vi "溶解氧电极校准.vi"() -> ()   [LabVIEW 2016, in "斯坦道多参数.lvlib"]
uses:
  <vilib>/Utility/miscctls.llb/LVPointTypeDef.ctl
  <vilib>/Analysis/NI_AALBase.lvlib
panel:
  out "第二点校准值":dbl
  out "第一点校准值":dbl
  out "最小值":sgl format="%#.2f"
  out "最大值":sgl format="%#.2f"
  in  "校准模式":enum16{"两点校准", "单点校准"}(ring)=enum."单点校准"
  in  "校准停止":bool
  in  "校准启动":bool
  out "波形图表":sgl(graph) caption="历史曲线"
  out "变异系数":dbl format="%#.6f"
  out "standard deviation":dbl caption="标准差" format="%#.2f"
  out "mean":dbl caption="均值" format="%#.2f"
  out "测量读值":dbl
  out "偏移值补偿":dbl
  out "饱和度值":dbl
  out "提示":string
  out "气压补偿值":dbl
  out "盐度补偿值":dbl
  out "电极斜率":dbl
  out "电极零点":dbl
  # "溶解氧电极设定"
  # "%"
  # "%"
  # "%"
  # "mg/L"
  # "ppt"
  # "hPa"
  # "mg/L"
  # "请选择校准模式:"
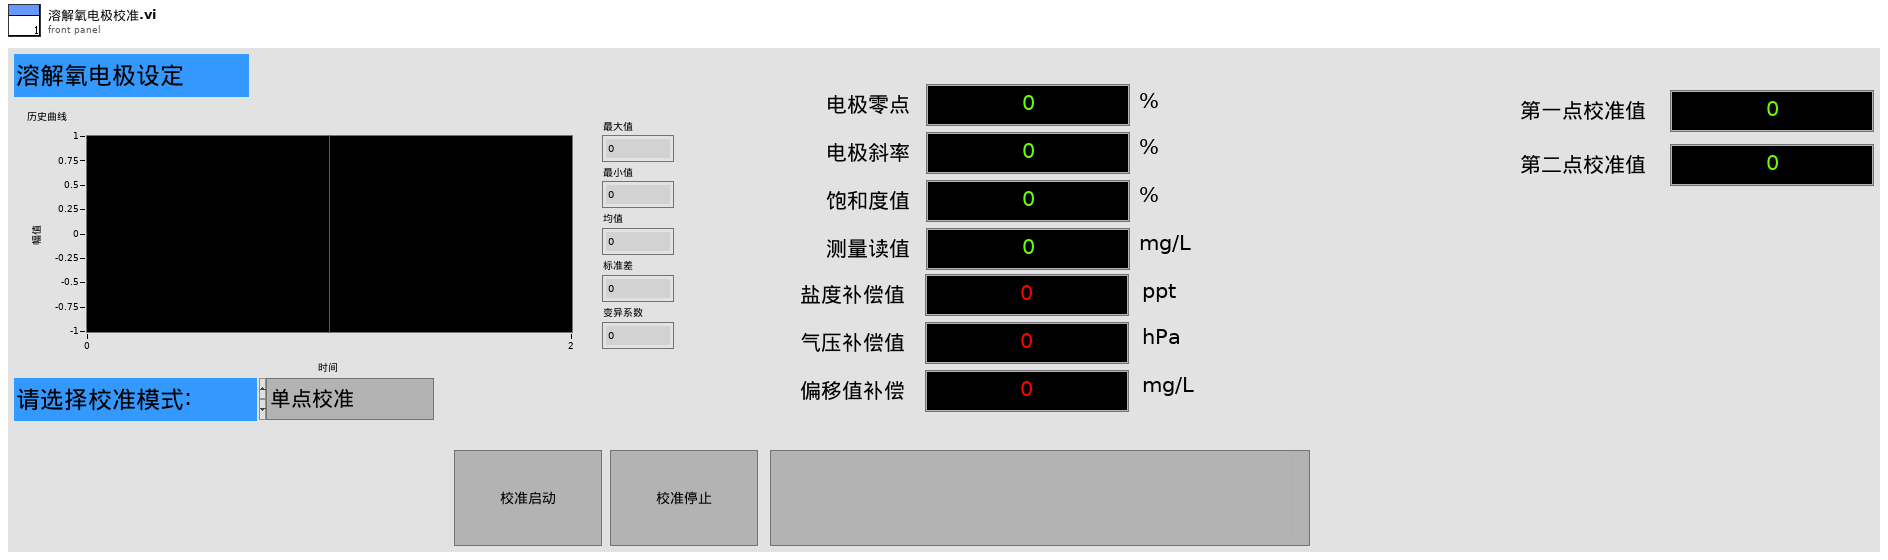
[diagram p1: front panel]
types:
  T1 = typedef "斯坦道多参数.lvlib/校准步骤.ctl" = enum16{"待机", "放置第一点标液", "第一点校准启动", "第一点校准写入", "第一点校准失败", "放置第二点标液", "第二点校准启动", "第二点校准写入", "第二点校准失败", "放置第三点标液", "第三点校准启动", "第三点校准写入", "第三点校准失败", "校准结果写入", "校准结束"}
  T2 = typedef "LVPointTypeDef.ctl" = cluster{"Horizontal":i16, "Vertical":i16}
  T3 = cluster{"电极状态标志":u16, "电极型号标志":u16, "溶解氧测量值":sgl, "温度测量值":sgl, "溶解氧饱和度值":sgl, "盐度补偿值":sgl, "大气压补偿值":sgl, "溶解氧偏移修正值":sgl, "温度偏移修正值":sgl, "手动温度补偿值":sgl, "溶解氧电极零点":sgl, "溶解氧电极斜率":sgl, "第1点标准值记录":sgl, "第1点信号值记录":sgl, "第1点温度值记录":sgl, "第2点标准值记录":sgl, "第2点信号值记录":sgl, "第2点温度值记录":sgl, "命令滤波设定":u16, "温度模式":enum16{"ATC", "MTC"}, "生产批次":u16, "电极序号":u16, "串口地址":u16, "串口波特率":enum16{"9600", "19200", "115200"}, "串口校验位":enum16{"NONE", "ODD", "EVEN"}, "串口停止位":enum16{"1bit", "2bit"}, "第一点标准值":sgl, "第二点标准值":sgl}
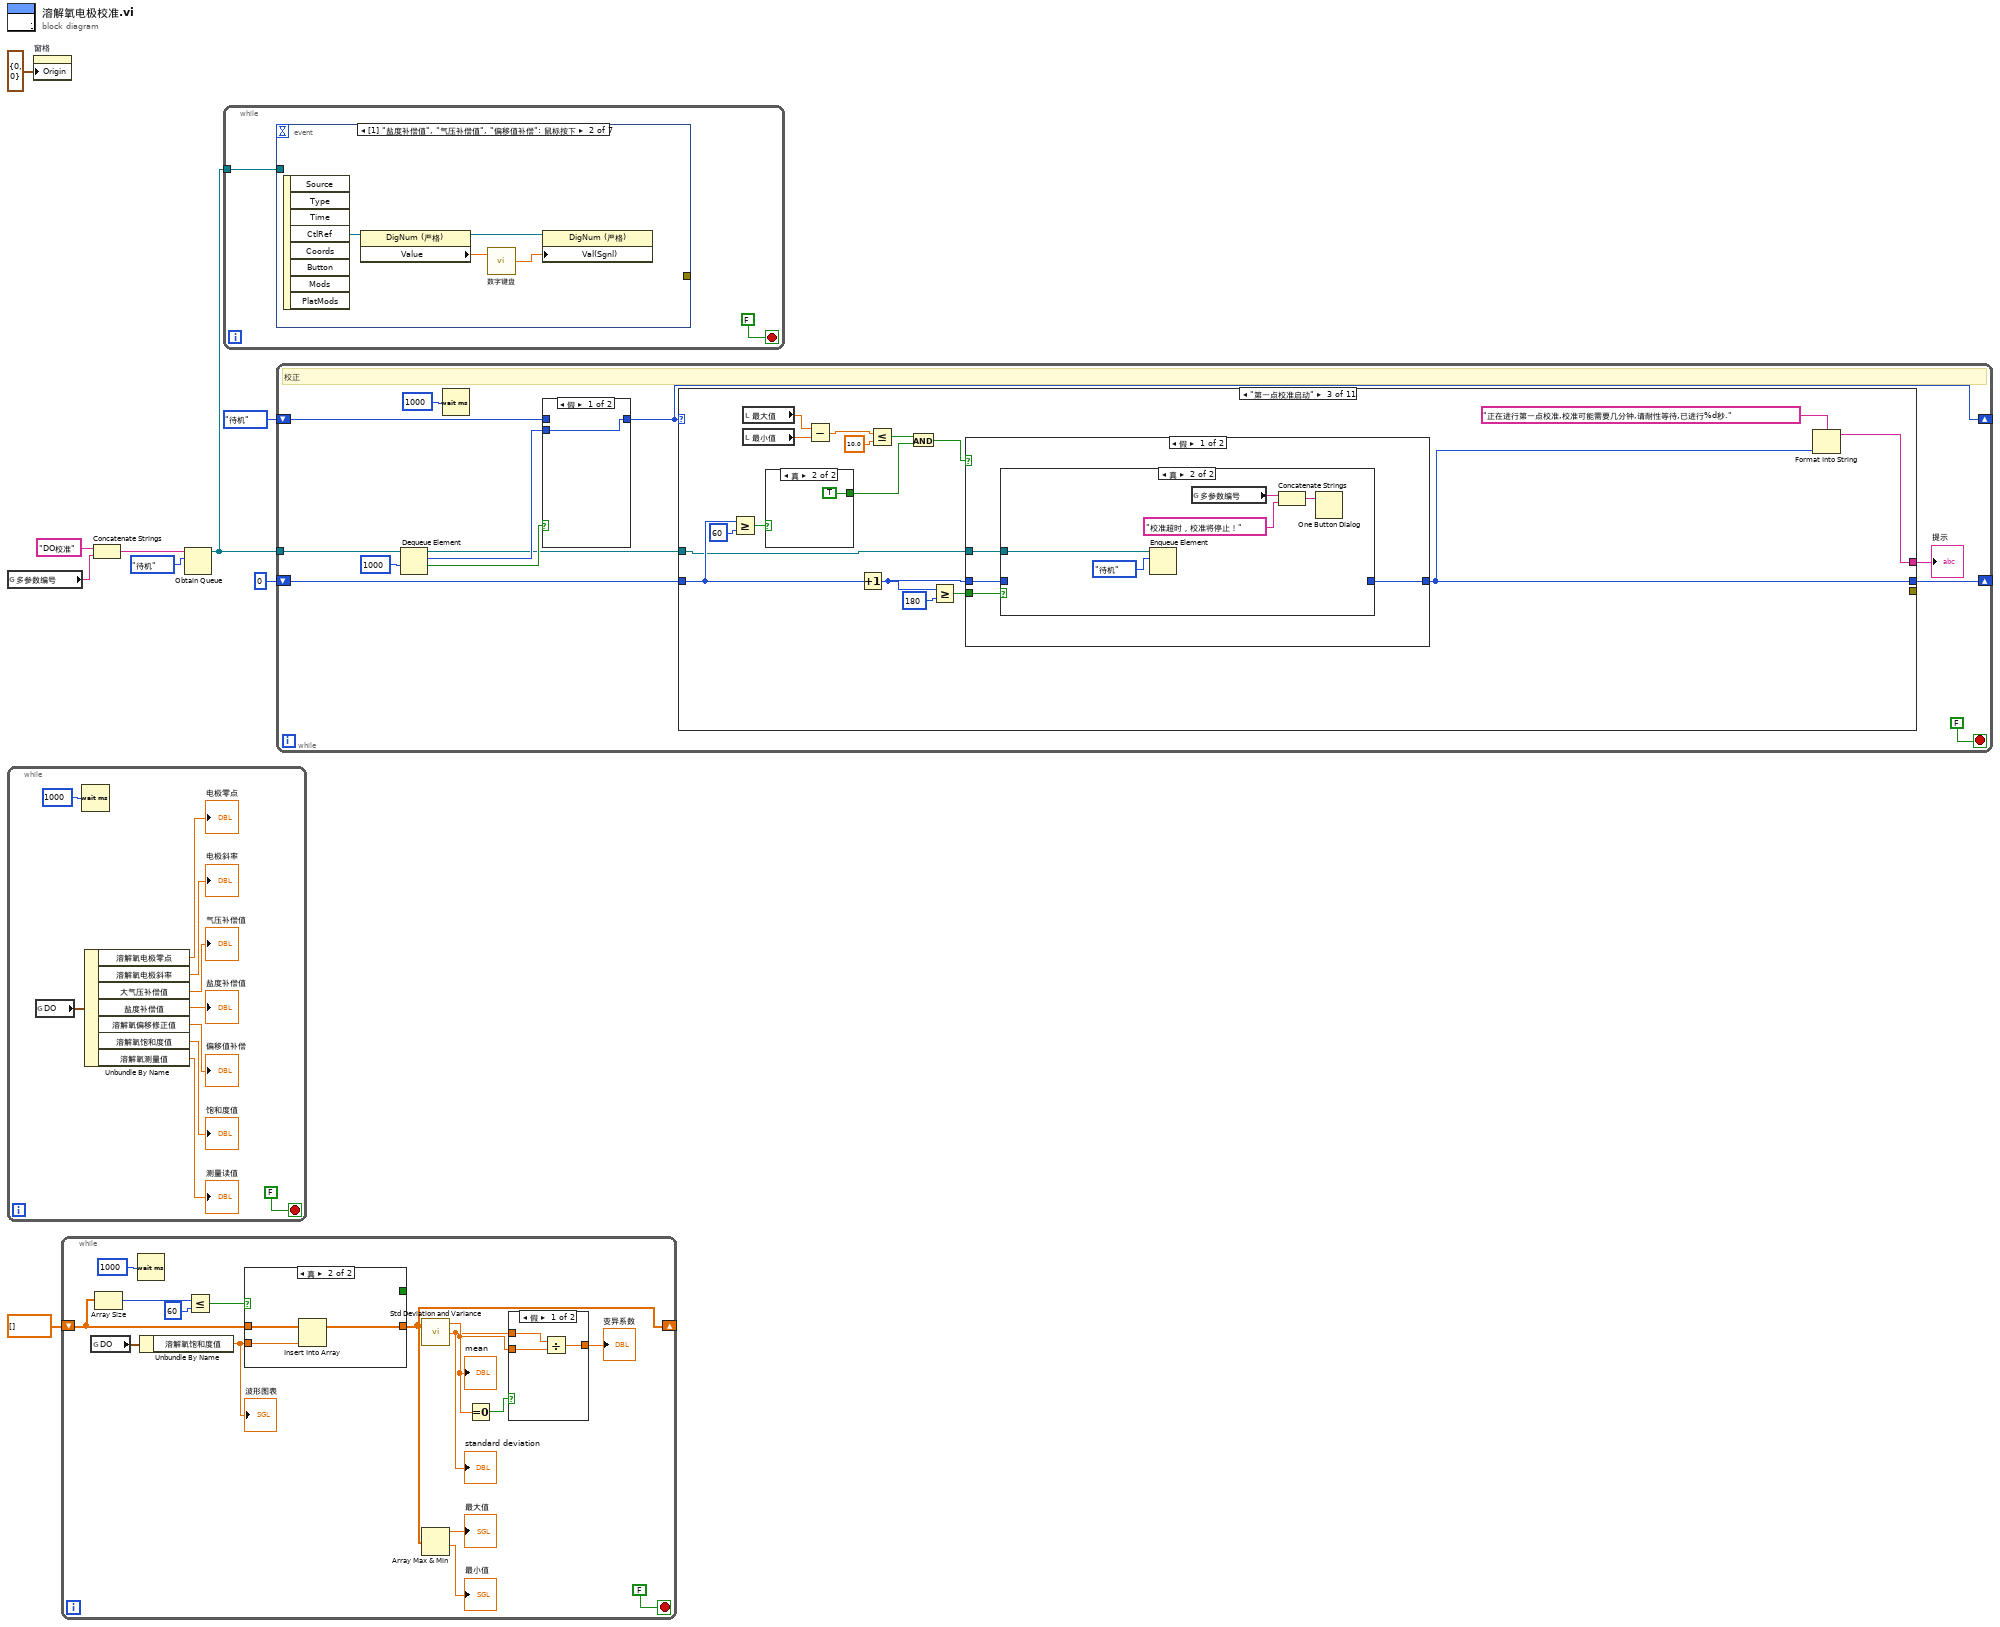
[diagram p0: block diagram]
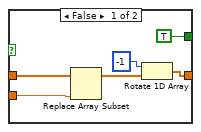
[diagram p3: hidden frame]
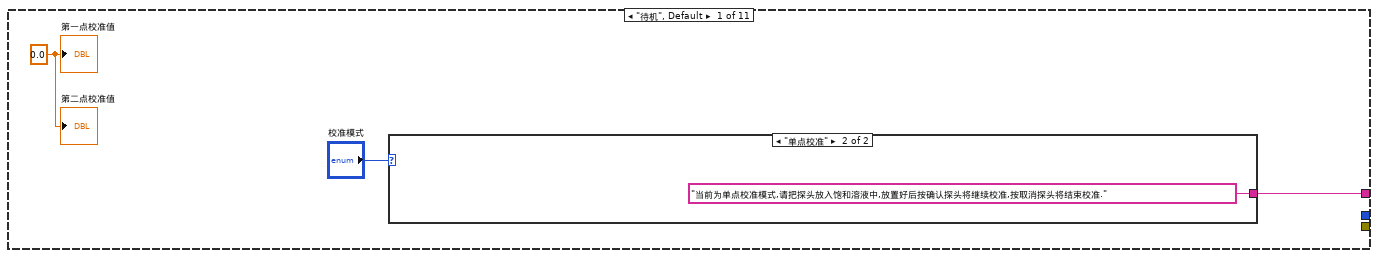
[diagram p5: hidden frame]
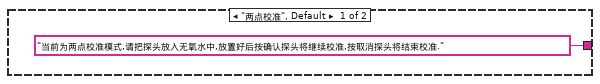
[diagram p6: hidden frame]
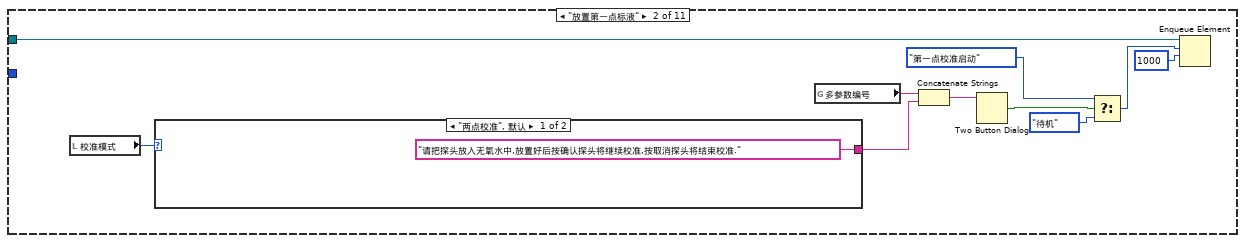
[diagram p7: hidden frame]
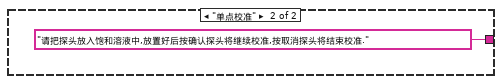
[diagram p8: hidden frame]
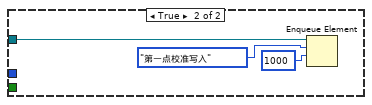
[diagram p10: hidden frame]
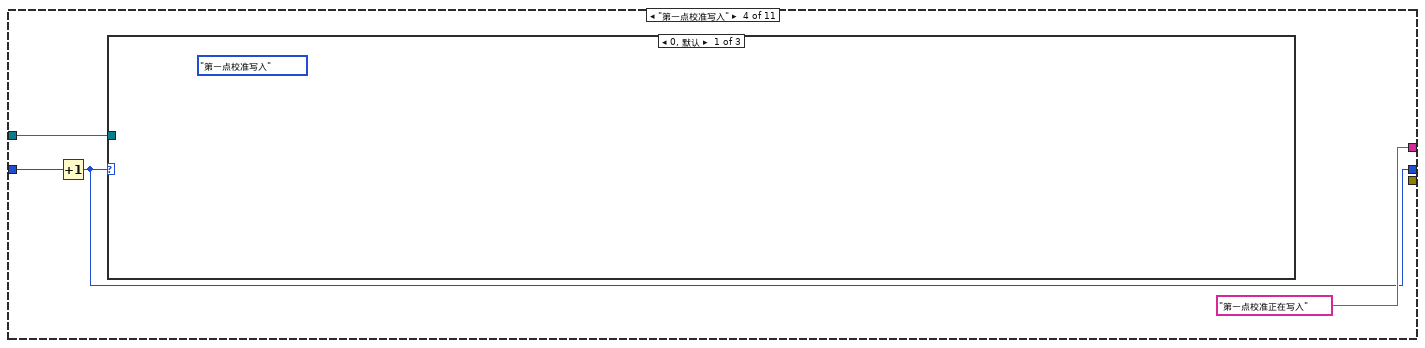
[diagram p12: hidden frame]
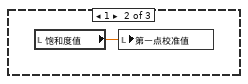
[diagram p13: hidden frame]
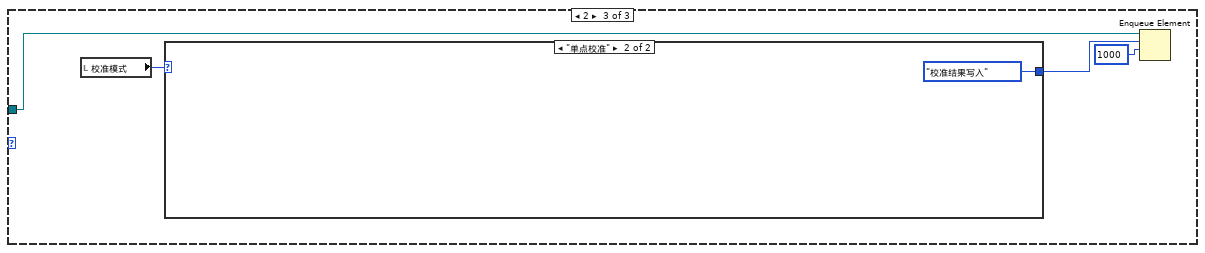
[diagram p14: hidden frame]
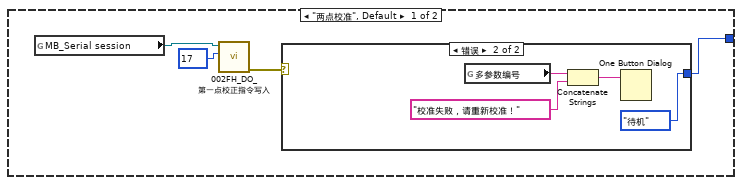
[diagram p15: hidden frame]
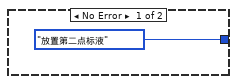
[diagram p16: hidden frame]
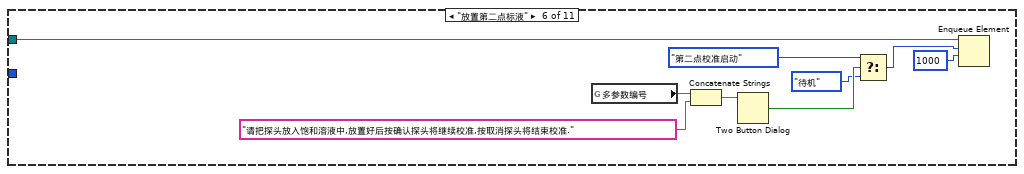
[diagram p18: hidden frame]
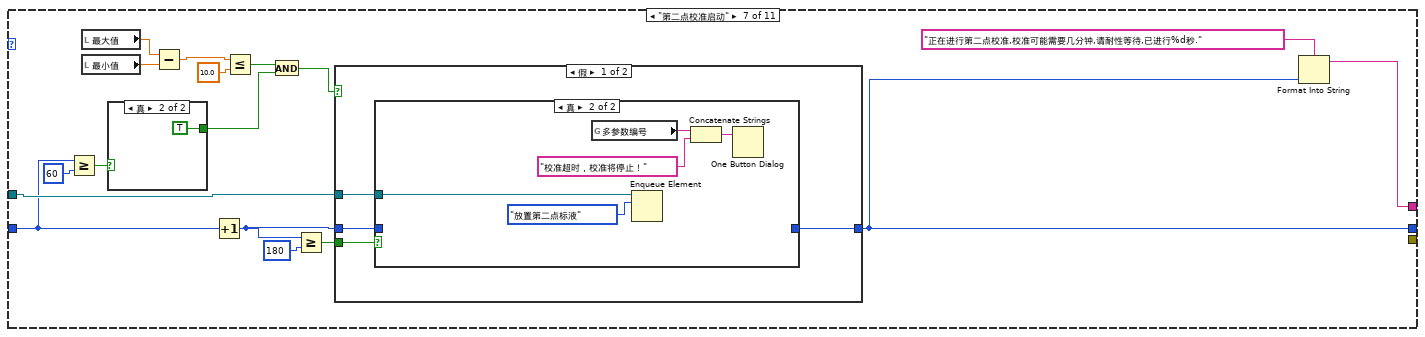
[diagram p19: hidden frame]
diagram:
  n1 = global read "多参数全局变量.vi" "多参数编号"() -> (w1:string)
  n2 = while {
    stop <- FALSE stop-if-true
    n3 = global read "国弘过程全局变量.vi" "DO"() -> (w17:T3)
    n4 = Wait (ms)(milliseconds to wait=u32 1000 ("等待时间（毫秒）")) -> ()  [unwired: 1 out]
    n5 = Unbundle By Name(w17) -> ("溶解氧电极零点"=→"电极零点":sgl, "溶解氧电极斜率"=→"电极斜率":sgl, "大气压补偿值"=→"气压补偿值":sgl, "盐度补偿值"=→"盐度补偿值":sgl, "溶解氧偏移修正值"=→"偏移值补偿":sgl, "溶解氧饱和度值"=→"饱和度值":sgl, "溶解氧测量值"=→"测量读值":sgl)
  }
  n6 = property on="窗格" class="Pane"("Origin"=T2 {"Horizontal"=0, "Vertical"=0} ("原点")) -> ()  [unwired: 2 in, 2 out]
  n7 = while {
    shift-right: [w23] -> _
    shift-left: sgl[] [] -> [w30]
    stop <- FALSE stop-if-true
    n8 = global read "国弘过程全局变量.vi" "DO"() -> (w26:T3)
    n9 = Array Size(array=w30) -> (size(s)=w32:i32)
    n10 = Wait (ms)(milliseconds to wait=u32 1000 ("等待时间（毫秒）")) -> ()  [unwired: 1 out]
    n11 = Unbundle By Name(w26) -> ("溶解氧饱和度值"=w20:sgl)
    "波形图表" <- w20
    n12 = Less Or Equal?(x=w32, y=60) -> (x <= y?=w31:bool)
    n13 = case shown="真" w31 {
      tunnel: w30 -> [w43 w46]
      tunnel: w20 -> [w41 w45]
      tunnel: [w39 w44] -> w23
      tunnel: [TRUE _] -> _
      frame False {
        n14 = Replace Array Subset(array=w43, new element=w41) -> (w42:sgl[])  [unwired: 1 in]
        n15 = Rotate 1D Array(1:w42, 2:-1 ("n")) -> (0:w39:sgl[])
      }
      frame True {
        n16 = Insert Into Array(array=w46, new element=w45) -> (w44:sgl[])  [unwired: 1 in]
      }
    }
    n17 = call <vilib>:"Std Deviation and Variance.vi"("X"=w23) -> ("mean"=w25:dbl, "standard deviation"=w24:dbl)  [unwired: 1 in, 1 out]
    "mean" <- w25
    "standard deviation" <- w24
    n18 = Array Max & Min(array=w23) -> (max value=→"最大值":sgl, min value=→"最小值":sgl)  [unwired: 2 out]
    n19 = Equal To 0?(x=w25) -> (x = 0?=w29:bool)
    n20 = case shown="假" w29 {
      tunnel: w24 -> [w37 _]
      tunnel: [w36 _] -> w28
      tunnel: w25 -> [w35 _]
      frame False {
        n21 = Divide(x=w37, y=w35) -> (x/y=w36:dbl)
      }
      frame True {
      }
    }
    "变异系数" <- w28
  }
  n22 = Concatenate Strings("DO校准" ("名称（未命名）"), w1) -> (w2:string)
  n23 = Obtain Queue(name (unnamed)=w2, element data type=校准步骤."待机" ("枚举")) -> (queue out=w3:refnum<queue>)  [unwired: 3 in, 2 out]
  n24 = while {
    tunnel: w3 -> [w47]
    stop <- FALSE stop-if-true
    n25 = event shown="[1] \"盐度补偿值\", \"气压补偿值\", \"偏移值补偿\": 鼠标按下" {
      selector: _ -> [_ _ _ _ _ _ _]
      dyn-events: _ -> [_ _ _ _ _ _ _]
      timeout: _ -> [_ _ _ _ _ _ _]
      tunnel: [_ _ w54 w57 w60 _ _] -> _
      tunnel: w47 -> [_ _ _ _ _ w62 w64]
      event Timeout {
        n26 = event-data() -> ()  [unwired: 1 in, 3 out]
      }
      event "盐度补偿值", "气压补偿值", "偏移值补偿": Mouse Down {
        n27 = event-data() -> ("CtlRef"=w50:refnum<vi>)  [unwired: 1 in, 7 out]
        n28 = property class="DigNum (严格)"(reference=w50) -> (reference out=w49:refnum<vi>, "Value"=w51:dbl)  [unwired: 1 in, 1 out]
        n29 = call "数字键盘.vi"("OldNumber"=w51) -> ("NewNumber"=w52:dbl)  [unwired: 1 in]
        n30 = property class="DigNum (严格)"(reference=w49, "Val(Sgnl)"=w52) -> ()  [unwired: 1 in, 2 out]
      }
      event "盐度补偿值": Value Change {
        n31 = event-data() -> ("NewVal"=w55:dbl)  [unwired: 1 in, 5 out]
        n32 = global read "多参数全局变量.vi" "MB_Serial session"() -> (w53:refnum<class "MB_Master_Serial.lvclass">)
        n33 = call "0008H_DO_盐度补偿值写入.vi"("数值"=w55, "MB_Serial session in"=w53) -> ("error out"=w54:errorcluster)  [unwired: 8 in, 1 out]
      }
      event "气压补偿值": Value Change {
        n34 = event-data() -> ("NewVal"=w58:dbl)  [unwired: 1 in, 5 out]
        n35 = global read "多参数全局变量.vi" "MB_Serial session"() -> (w56:refnum<class "MB_Master_Serial.lvclass">)
        n36 = call "000AH_DO_大气压补偿值写入.vi"("数值"=w58, "MB_Serial session in"=w56) -> ("error out"=w57:errorcluster)  [unwired: 8 in, 1 out]
      }
      event "偏移值补偿": Value Change {
        n37 = event-data() -> ("NewVal"=w61:dbl)  [unwired: 1 in, 5 out]
        n38 = global read "多参数全局变量.vi" "MB_Serial session"() -> (w59:refnum<class "MB_Master_Serial.lvclass">)
        n39 = call "000CH_DO_DO偏移修正值写入.vi"("数值"=w61, "MB_Serial session in"=w59) -> ("error out"=w60:errorcluster)  [unwired: 8 in, 1 out]
      }
      event "校准启动": Value Change {
        n40 = event-data() -> ()  [unwired: 1 in, 6 out]
        n41 = Enqueue Element(queue=w62, element=校准步骤."放置第一点标液" ("元素")) -> ()  [unwired: 2 in, 3 out]
      }
      event "校准停止": Value Change {
        n42 = event-data() -> ()  [unwired: 1 in, 6 out]
        n43 = Flush Queue(queue=w64) -> (queue out=w65:refnum<queue>)  [unwired: 1 in, 2 out]
        n44 = Enqueue Element(queue=w65, element=校准步骤."待机" ("元素"), timeout in ms (-1)=1000 ("超时毫秒(-1)")) -> ()  [unwired: 1 in, 3 out]
      }
    }
  }
  n45 = while "While循环" {
    shift-right: [w69] -> _
    shift-left: 校准步骤."待机" ("枚举") -> [w70]
    shift-right: [w76] -> _
    shift-left: 0 -> [w77]
    tunnel: w3 -> [w71]
    stop <- FALSE stop-if-true
    # "校正"
    n46 = Dequeue Element(queue=w71, timeout in ms (-1)=1000 ("超时毫秒(-1)")) -> (queue out=w68:refnum<queue>, element=w72:T1, timed out?=w73:bool)  [unwired: 1 in, 1 out]
    n47 = Wait (ms)(milliseconds to wait=u32 1000 ("等待时间（毫秒）")) -> ()  [unwired: 1 out]
    n48 = case shown="假" w73 {
      tunnel: w72 -> [w80 _]
      tunnel: [w80 w81] -> w69
      tunnel: w70 -> [_ w81]
      frame False {
      }
      frame True {
      }
    }
    n49 = case shown="\"第一点校准启动\"" w69 {
      tunnel: [w84 _ w103 "第一点校准正在写入" ("提示") _ _ w159 "第二点校准正在写入" ("提示") _ w206 w236] -> w75
      tunnel: w77 -> [_ _ w107 w132 _ _ w161 w191 _ _ _]
      tunnel: [_ _ w106 w131 _ _ w160 w190 _ _ _] -> w76
      tunnel: w68 -> [_ w90 w105 w130 _ w151 w162 w189 _ w210 _]
      tunnel: [_ _ _ _ _ _ _ _ _ w205 _] -> _
      frame "待机", Default {
        w82 = 0.0 ("第一点校准值")
        n50 = case shown="\"单点校准\"" "校准模式" {
          tunnel: ["当前为两点校准模式,请把探头放入无氧水中,放置好后按确认探头将继续校准,按取消探头将结束校准." ("消息") "当前为单点校准模式,请把探头放入饱和溶液中,放置好后按确认探头将继续校准,按取消探头将结束校准." ("消息")] -> w84
          frame "两点校准", Default {
          }
          frame "单点校准" {
          }
        }
        "第一点校准值" <- w82
        "第二点校准值" <- w82
      }
      frame "放置第一点标液" {
        n51 = local read "校准模式"() -> (w89:enum16{"两点校准", "单点校准"})
        n52 = case shown="\"两点校准\", 默认" w89 {
          tunnel: ["请把探头放入无氧水中,放置好后按确认探头将继续校准,按取消探头将结束校准." ("消息") "请把探头放入饱和溶液中,放置好后按确认探头将继续校准,按取消探头将结束校准." ("消息")] -> w96
          frame "两点校准", Default {
          }
          frame "单点校准" {
          }
        }
        n53 = global read "多参数全局变量.vi" "多参数编号"() -> (w87:string)
        n54 = Concatenate Strings(w87, w96) -> (w88:string)
        n55 = Two Button Dialog(message=w88) -> (T button?=w94:bool)  [unwired: 2 in]
        n56 = Select(t=校准步骤."第一点校准启动" ("元素"), s=w94, f=校准步骤."待机" ("元素")) -> (s? t:f=w91:T1)
        n57 = Enqueue Element(queue=w90, element=w91, timeout in ms (-1)=1000 ("超时毫秒(-1)")) -> ()  [unwired: 1 in, 3 out]
      }
      frame "第一点校准启动" {
        n58 = Greater Or Equal?(x=w107, y=60) -> (x >= y?=w114:bool)
        n59 = local read "最大值"() -> (w111:sgl)
        n60 = local read "最小值"() -> (w110:sgl)
        n61 = case shown="真" w114 {
          tunnel: [_ TRUE] -> w102
          frame False {
          }
          frame True {
          }
        }
        n62 = Subtract(x=w111, y=w110) -> (x-y=w112:sgl)
        n63 = Increment(x=w107) -> (x+1=w104:i32)
        n64 = Less Or Equal?(x=w112, y=10.0) -> (x <= y?=w101:bool)
        n65 = And(x=w101, y=w102) -> (x .and. y?=w100:bool)
        n66 = Greater Or Equal?(x=w104, y=180) -> (x >= y?=w108:bool)
        n67 = case shown="假" w100 {
          tunnel: w105 -> [w118 w128]
          tunnel: w108 -> [w119 _]
          tunnel: w104 -> [w117 _]
          tunnel: [w116 _] -> w106
          frame False {
            n68 = case shown="真" w119 {
              tunnel: w118 -> [_ w125]
              tunnel: w117 -> [w120 _]
              tunnel: [w120 _] -> w116
              frame False {
              }
              frame True {
                n69 = Enqueue Element(queue=w125, element=校准步骤."待机" ("元素")) -> ()  [unwired: 2 in, 3 out]
                n70 = global read "多参数全局变量.vi" "多参数编号"() -> (w121:string)
                n71 = Concatenate Strings(w121, "校准超时，校准将停止！" ("消息")) -> (w122:string)
                n72 = One Button Dialog(message=w122) -> ()  [unwired: 1 in, 1 out]
              }
            }
          }
          frame True {
            n73 = Enqueue Element(queue=w128, element=校准步骤."第一点校准写入" ("元素"), timeout in ms (-1)=1000 ("超时毫秒(-1)")) -> ()  [unwired: 1 in, 3 out]
          }
        }
        n74 = Format Into String(format string="正在进行第一点校准,校准可能需要几分钟,请耐性等待,已进行%d秒." ("格式字符串"), w106) -> (resulting string=w103:string)  [unwired: 2 in, 1 out]
      }
      frame "第一点校准写入" {
        n75 = Increment(x=w132) -> (x+1=w131:i32)
        n76 = case shown="0, 默认" w131 {
          tunnel: w130 -> [_ _ w136]
          frame 0, Default {
            (unwired) 校准步骤."第一点校准写入" ("枚举")
          }
          frame 1 {
            n77 = local read "饱和度值"() -> (w134:dbl)
            n78 = local write "第一点校准值"(w134) -> ()
          }
          frame 2 {
            n79 = local read "校准模式"() -> (w138:enum16{"两点校准", "单点校准"})
            n80 = case shown="\"单点校准\"" w138 {
              tunnel: [w139 校准步骤."校准结果写入" ("枚举")] -> w135
              frame "两点校准", Default {
                n81 = global read "多参数全局变量.vi" "MB_Serial session"() -> (w140:refnum<class "MB_Master_Serial.lvclass">)
                n82 = call "002FH_DO_第一点校正指令写入.vi"("数值"=u16 17, "MB_Serial session in"=w140) -> ("error out"=w141:errorcluster)  [unwired: 8 in, 1 out]
                n83 = case shown="错误" w141 {
                  tunnel: [校准步骤."放置第二点标液" ("元素") 校准步骤."待机" ("元素")] -> w139
                  frame No Error {
                  }
                  frame Error {
                    n84 = global read "多参数全局变量.vi" "多参数编号"() -> (w144:string)
                    n85 = Concatenate Strings(w144, "校准失败，请重新校准！" ("消息")) -> (w145:string)
                    n86 = One Button Dialog(message=w145) -> ()  [unwired: 1 in, 1 out]
                  }
                }
              }
              frame "单点校准" {
              }
            }
            n87 = Enqueue Element(queue=w136, element=w135, timeout in ms (-1)=1000 ("超时毫秒(-1)")) -> ()  [unwired: 1 in, 3 out]
          }
        }
      }
      frame "第一点校准失败" {
      }
      frame "放置第二点标液" {
        n88 = global read "多参数全局变量.vi" "多参数编号"() -> (w149:string)
        n89 = Concatenate Strings(w149, "请把探头放入饱和溶液中,放置好后按确认探头将继续校准,按取消探头将结束校准." ("消息")) -> (w150:string)
        n90 = Two Button Dialog(message=w150) -> (T button?=w155:bool)  [unwired: 2 in]
        n91 = Select(t=校准步骤."第二点校准启动" ("元素"), s=w155, f=校准步骤."待机" ("元素")) -> (s? t:f=w152:T1)
        n92 = Enqueue Element(queue=w151, element=w152, timeout in ms (-1)=1000 ("超时毫秒(-1)")) -> ()  [unwired: 1 in, 3 out]
      }
      frame "第二点校准启动" {
        n93 = Greater Or Equal?(x=w161, y=60) -> (x >= y?=w173:bool)
        n94 = local read "最大值"() -> (w170:sgl)
        n95 = local read "最小值"() -> (w169:sgl)
        n96 = case shown="真" w173 {
          tunnel: [_ TRUE] -> w166
          frame False {
          }
          frame True {
          }
        }
        n97 = Subtract(x=w170, y=w169) -> (x-y=w171:sgl)
        n98 = Increment(x=w161) -> (x+1=w167:i32)
        n99 = Less Or Equal?(x=w171, y=10.0) -> (x <= y?=w165:bool)
        n100 = And(x=w165, y=w166) -> (x .and. y?=w164:bool)
        n101 = Greater Or Equal?(x=w167, y=180) -> (x >= y?=w168:bool)
        n102 = case shown="假" w164 {
          tunnel: w162 -> [w177 w187]
          tunnel: w168 -> [w178 _]
          tunnel: w167 -> [w176 _]
          tunnel: [w175 _] -> w160
          frame False {
            n103 = case shown="真" w178 {
              tunnel: w177 -> [_ w184]
              tunnel: w176 -> [w179 _]
              tunnel: [w179 _] -> w175
              frame False {
              }
              frame True {
                n104 = global read "多参数全局变量.vi" "多参数编号"() -> (w180:string)
                n105 = Enqueue Element(queue=w184, element=校准步骤."放置第二点标液" ("元素")) -> ()  [unwired: 2 in, 3 out]
                n106 = Concatenate Strings(w180, "校准超时，校准将停止！" ("消息")) -> (w182:string)
                n107 = One Button Dialog(message=w182) -> ()  [unwired: 1 in, 1 out]
              }
            }
          }
          frame True {
            n108 = Enqueue Element(queue=w187, element=校准步骤."第二点校准写入" ("元素"), timeout in ms (-1)=1000 ("超时毫秒(-1)")) -> ()  [unwired: 1 in, 3 out]
          }
        }
        n109 = Format Into String(format string="正在进行第二点校准,校准可能需要几分钟,请耐性等待,已进行%d秒." ("格式字符串"), w160) -> (resulting string=w159:string)  [unwired: 2 in, 1 out]
      }
      frame "第二点校准写入" {
        n110 = Increment(x=w191) -> (x+1=w190:i32)
        n111 = case shown="0, 默认" w190 {
          tunnel: w189 -> [_ _ w194]
          frame 0, Default {
            (unwired) 校准步骤."第二点校准写入" ("枚举")
          }
          frame 1 {
            n112 = local read "饱和度值"() -> (w193:dbl)
            n113 = local write "第二点校准值"(w193) -> ()
          }
          frame 2 {
            n114 = global read "多参数全局变量.vi" "MB_Serial session"() -> (w198:refnum<class "MB_Master_Serial.lvclass">)
            n115 = call "0032H_DO_第二点校正指令写入.vi"("数值"=u16 33, "MB_Serial session in"=w198) -> ("error out"=w195:errorcluster)  [unwired: 8 in, 1 out]
            n116 = case shown="错误" w195 {
              tunnel: [校准步骤."校准结果写入" ("元素") 校准步骤."放置第二点标液" ("元素")] -> w196
              frame No Error {
              }
              frame Error {
                n117 = global read "多参数全局变量.vi" "多参数编号"() -> (w201:string)
                n118 = Concatenate Strings(w201, "校准失败，请重新校准！" ("消息")) -> (w202:string)
                n119 = One Button Dialog(message=w202) -> ()  [unwired: 1 in, 1 out]
              }
            }
            n120 = Enqueue Element(queue=w194, element=w196, timeout in ms (-1)=1000 ("超时毫秒(-1)")) -> ()  [unwired: 1 in, 3 out]
          }
        }
      }
      frame "第二点校准失败" {
      }
      frame "校准结果写入" {
        n121 = Enqueue Element(queue=w210, element=校准步骤."校准结束" ("元素")) -> ()  [unwired: 2 in, 3 out]
        n122 = local read "校准模式"() -> (w209:enum16{"两点校准", "单点校准"})
        n123 = case shown="\"单点校准\"" w209 {
          tunnel: [w212 w228] -> w208
          frame "两点校准", Default {
            n124 = global read "国弘过程全局变量.vi" "DO"() -> (w214:T3)
            n125 = Unbundle By Name(w214) -> ("电极状态标志"=w213:u16)
            n126 = case shown="3, 4" w213 {
              selector: w213 -> [w216 _ w225]
              tunnel: [w215 w220 w224] -> w212
              frame 0, Default {
                n127 = case shown="1" w216 {
                  tunnel: ["校正未正常启动，请重新校正" "第一点校准通过" "第二点校准通过"] -> w215
                  frame 0, Default {
                  }
                  frame 1 {
                  }
                  frame 2 {
                  }
                }
              }
              frame 2 {
                n128 = local read "第一点校准值"() -> (w222:dbl)
                n129 = local read "第二点校准值"() -> (w223:dbl)
                n130 = Format Into String(format string="两点校准结果：第一点校准值：%f；第二点校准值：%f。" ("提示"), w222, w223) -> (resulting string=w220:string)  [unwired: 2 in, 1 out]
              }
              frame 3, 4 {
                n131 = case shown="4" w225 {
                  tunnel: ["校正失败，电极零点超出范围" "校正失败，电极斜率超出范围"] -> w224
                  frame 3, Default {
                  }
                  frame 4 {
                  }
                }
              }
            }
          }
          frame "单点校准" {
            n132 = global read "多参数全局变量.vi" "MB_Serial session"() -> (w230:refnum<class "MB_Master_Serial.lvclass">)
            n133 = call "0032H_DO_第二点校正指令写入.vi"("数值"=u16 33, "MB_Serial session in"=w230) -> ("error out"=w229:errorcluster)  [unwired: 8 in, 1 out]
            n134 = case shown="无错误" w229 {
              tunnel: [w232 "校准失败，请重新校准！" ("消息")] -> w228
              frame No Error {
                n135 = local read "第一点校准值"() -> (w233:dbl)
                n136 = Format Into String(format string="单点校准结果：校准值：%f" ("提示"), w233) -> (resulting string=w232:string)  [unwired: 2 in, 1 out]
              }
              frame Error {
              }
            }
          }
        }
        n137 = global read "多参数全局变量.vi" "多参数编号"() -> (w207:string)
        n138 = Concatenate Strings(w207, w208) -> (w206:string)
        n139 = One Button Dialog(message=w206) -> ()  [unwired: 1 in, 1 out]
        n140 = call "操作日志.vi"("日志信息"=w206) -> ("error out"=w205:errorcluster)  [unwired: 10 in]
      }
      frame "校准结束" {
        n141 = local read "提示"() -> (w236:string)
      }
    }
    "提示" <- w75
  }
